vi "ConvertCalibStuff.vi"(11 "Settings in":T2={"Name of test"="", "Date"=timestamp(0 s since 1904-01-01), "Location"="", "Template"="", "Soundcard"="", "resolution"=0, "Sampling rate"=0, "Ch1 Gain "=0.0, "Ch2 Gain"=0.0, "Sample time (s)"=0.0, "Pre-trigger (s)"=0.0, "Hammer Threshold"=0.0, "Positions"=0, "Taps/Position"=0, "Set Names"="", "Freq resolution"=0.0, "Hammer cutoff"=0.0, "Mic cutoff"=0.0, "Double bounce "=0.0, "Hammer Cal"=0.0, "dB Offset"=0.0, "Accel Cal"=0.0, "Vibrometer Cal"=0.0, "Mic Cal"=0.0, "Output"=0, "Voltage Cal"=0.0, "Vibrometer Port"="", "Range"=0, "High Pass"=0, "Bandwidth"=0, "X Range"=[], "Y Range"=[], "dB Spread"=0.0, "Trigger"=0, "Ch_1"=0, "Ch_2"=0, "flip?"=FALSE, "60Hz"=FALSE, "Time offset"=0.0, "Piezo Cal"=1.0, "Default Notes"="", "Tom"=FALSE} {"Ch_2" min=1 step=1; "Ch_1" min=1 max=100 step=1; "Trigger" items=["Hammer (force)", "Self-tap", "Spacebar"]; "Bandwidth" items=["1 kHz"=1, "5 kHz"=5, "10 kHz"=10, "25 kHz"=25, "50 kHz"=50, "100 kHz"=100]; "High Pass" items=["Off", "13 Hz", "104 Hz"]; "Range" items=["10 mm/s"=1, "20 mm/s"=2, "50 mm/s"=5, "100 mm/s"=10, "200 mm/s"=20, "500 mm/s"=50, "1 m/s"=100, "2 m/s"=200]; "Output" items=["Accelerometer", "Speed (from acceleration)", "Microphone", "Vibrometer", "Piezo"]; "Voltage Cal" format="%#_13g"; "Ch2 Gain" format="%#_13g"; "Ch1 Gain" format="%#_13g"; "Double bounce" min=0.0; "Mic cutoff" min=0.0 format="%#_4g"; "Hammer cutoff" min=0.0 format="%#_4g"; "Freq resolution" min=0.0; "Pre-trigger (s)" format="%#_13g"; "Date" format="%<%H:%M\n%d/%m/%y>T"; "resolution" items=["16 bit"=16, "24 bit"=24, "32 bit"=32]; "Sampling rate" items=["22050 samp/s"=22050, "44100 samp/s"=44100, "48000 samp/s"=48000]}) -> (1 "Text":string, 2 "cluster":T1, 3 "File":string, 5 "titles":string[](array[string])=["Voltage", "Microphone", "Accelerometer", "Vibrometer", "Hammer", "Flip"])   [LabVIEW 2022 SP3]
uses:
  PreferencesControl.ctl
panel:
  # "Hz"
  # "dB"
  # "dB"
  # "sec"
  # "sec"
  # "mV/Pa"
  # "mV/m/s2"
  # "mV/mm/s"
  # "V/N"
  # "sec"
  # "sec"
  # "mV/N"
  # "a.u."
  # "a.u."
  # "sec"
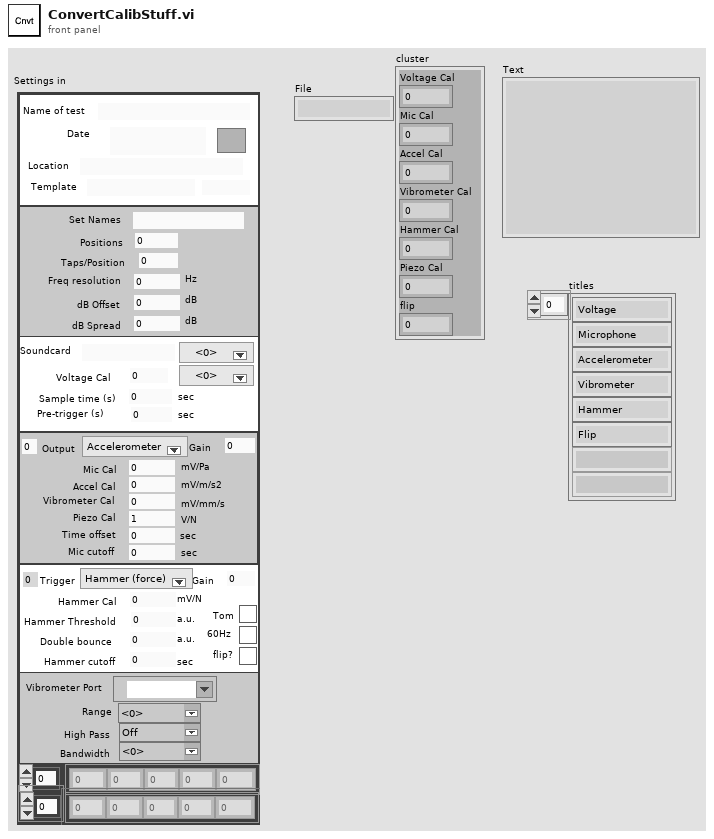
[diagram p1: front panel]
types:
  T1 = cluster{"Voltage Cal":dbl, "Mic Cal":dbl, "Accel Cal":dbl, "Vibrometer Cal":dbl, "Hammer Cal":dbl, "Piezo Cal":dbl, "flip":dbl}
  T2 = typedef "PreferencesControl.ctl" = cluster{"Name of test":string, "Date":timestamp, "Location":string, "Template":string, "Soundcard":string, "resolution":u16, "Sampling rate":u16, "Ch1 Gain ":dbl, "Ch2 Gain":dbl, "Sample time (s)":dbl, "Pre-trigger (s)":dbl, "Hammer Threshold":dbl, "Positions":i16, "Taps/Position":i16, "Set Names":string, "Freq resolution":dbl, "Hammer cutoff":dbl, "Mic cutoff":dbl, "Double bounce ":dbl, "Hammer Cal":dbl, "dB Offset":dbl, "Accel Cal":dbl, "Vibrometer Cal":dbl, "Mic Cal":dbl, "Output":u16, "Voltage Cal":dbl, "Vibrometer Port":refnum<visa-resource-name>, "Range":u16, "High Pass":u16, "Bandwidth":u16, "X Range":cluster{"Minimum":dbl, "Maximum":dbl, "Increment":dbl, "Minor Increment":dbl, "Start":dbl}[], "Y Range":cluster{"Minimum":dbl, "Maximum":dbl, "Increment":dbl, "Minor Increment":dbl, "Start":dbl}[], "dB Spread":dbl, "Trigger":u16, "Ch_1":u8, "Ch_2":u8, "flip?":bool, "60Hz":bool, "Time offset":dbl, "Piezo Cal":dbl, "Default Notes":string, "Tom":bool}
  T3 = cluster{"Voltage Cal":dbl, "Mic Cal":dbl, "Accel Cal":dbl, "Vibrometer Cal":dbl, "Hammer Cal":dbl, "Piezo Cal":dbl, dbl}
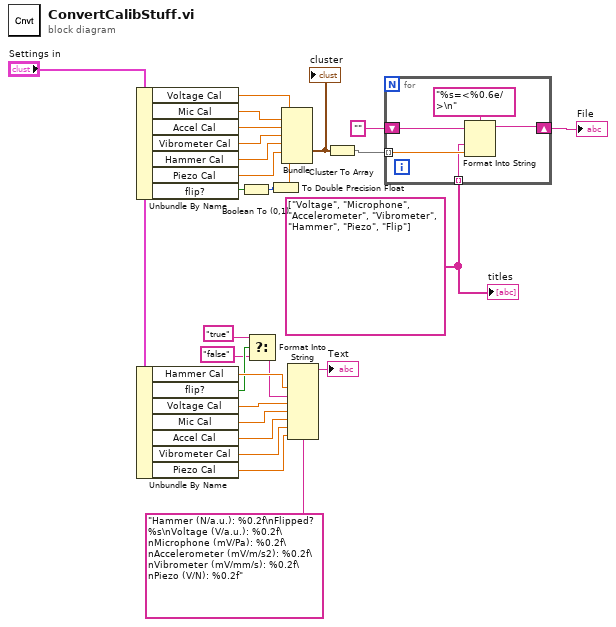
[diagram p0: block diagram]
diagram:
  w16 = string[] ["Voltage", "Microphone", "Accelerometer", "Vibrometer", "Hammer", "Piezo", "Flip"]
  n1 = Unbundle By Name("Settings in") -> ("Voltage Cal"=w21:dbl, "Mic Cal"=w20:dbl, "Accel Cal"=w19:dbl, "Vibrometer Cal"=w18:dbl, "Hammer Cal"=w17:dbl, "Piezo Cal"=w2:dbl, "flip?"=w26:bool)
  n2 = Unbundle By Name("Settings in") -> ("Hammer Cal"=w14:dbl, "flip?"=w8:bool, "Voltage Cal"=w13:dbl, "Mic Cal"=w12:dbl, "Accel Cal"=w11:dbl, "Vibrometer Cal"=w10:dbl, "Piezo Cal"=w1:dbl)
  n3 = Boolean To (0,1)(Boolean=w26) -> (0, 1=w25:i16)
  n4 = Select(t="true" ("format string"), s=w8, f="false" ("format string")) -> (s? t:f=w6:string)
  n5 = To Double Precision Float(number=w25) -> (double precision float=w3:dbl)
  n6 = Bundle("Voltage Cal"=w21, "Mic Cal"=w20, "Accel Cal"=w19, "Vibrometer Cal"=w18, "Hammer Cal"=w17, "Piezo Cal"=w2, w3) -> (w22:T3)  [unwired: 1 in]
  "cluster" <- w22
  n7 = Format Into String(format string="Hammer (N/a.u.): %0.2f\nFlipped? %s\nVoltage (V/a.u.): %0.2f\nMicrophone (mV/Pa): %0.2f\nAccelerometer (mV/m/s2): %0.2f\nVibrometer (mV/mm/s): %0.2f\nPiezo (V/N): %0.2f", w14, w6, w13, w12, w11, w10, w1) -> (resulting string=→"Text":string)  [unwired: 2 in, 1 out]
  n8 = Cluster To Array(cluster=w22) -> (array=w23:dbl[])
  n9 = for {
    tunnel: w23 -> [w31] mode=indexing
    tunnel: w16 -> [w30] mode=indexing
    shift-right: [w28] -> w27
    shift-left: "" -> [w29]
    n10 = Format Into String(format string="%s=<%0.6e/>\n", initial string=w29, w30, w31) -> (resulting string=w28:string)  [unwired: 1 in, 1 out]
  }
  "File" <- w27
  "titles" <- w16
